vi "Report Plotter.vi"(0 "Plot":refnum<vi>, 1 "Path":refnum<vi>, 2 "Vision Overlay":refnum<vi>, 3 "Indicators":T2, 4 "Play":refnum<vi>, 5 "Exit":refnum<vi>, 7 "Visualized Color Plane":refnum<vi>, 9 "Slider":refnum<vi>, 11 "error in":errorcluster, 12 "Image Indicator":variant, 13 "Loading Bar":refnum<vi>, 14 "Image Type":T1=4 items=["Grayscale (U8)", "Grayscale (I16)", "Grayscale (SGL)", "Complex (CSG)", "RGB (U32)", "HSL (U32)", "RGB (U64)", "Grayscale (U16)"]) -> (15 "error out":errorcluster)   [LabVIEW 2012, in "Report.lvlib"]
uses:
  Report.lvlib
  <vilib>/Waveform/WDTOps.llb/WDT Get XY Value DBL.vi
  <vilib>/Waveform/WDTOps.llb/WDT Number of Waveform Samples DBL.vi
  <vilib>/Utility/xml.llb/Read From XML File(array).vi
  <vilib>/vision/NI_Vision_Development_Module.lvlib
panel:
  out "XML Elements":string[](array[string])
  out "Exit":bool
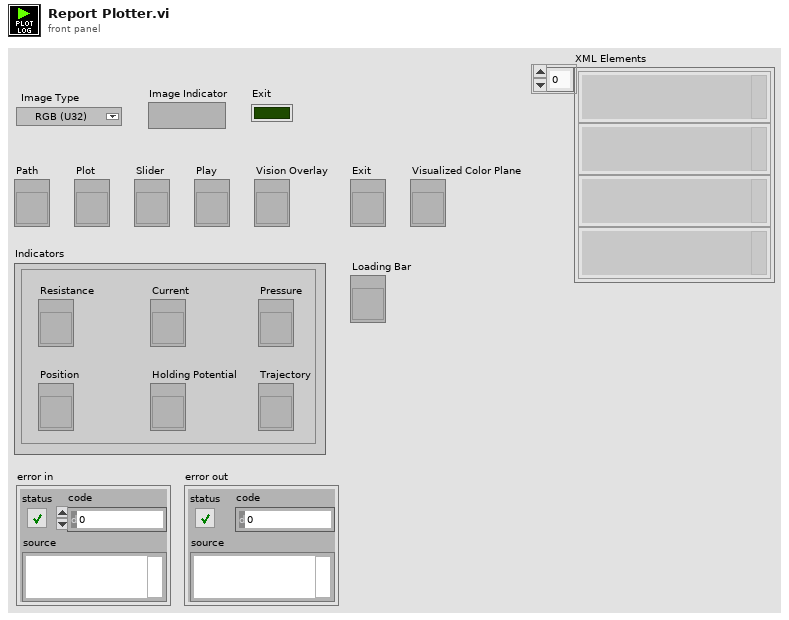
[diagram p1: front panel]
types:
  T1 = typedef "Image Type" = u32
  T2 = cluster{"Resistance":refnum<vi>, "Current":refnum<vi>, "Pressure":refnum<vi>, "Holding Potential":refnum<vi>, "Position":refnum<vi>, "Trajectory":refnum<vi>}
  T3 = cluster{"Name":string, "Color":u32, "Style":u8, "Point Style":u8, "Name Visible":bool, "Allow Drag":bool, "Cursor Mode":u32, "Plot":i32, "Index":i32, "Position":cluster{"X":dbl, "Y":dbl}, "X Scale":u32, "Y Scale":u32, "Watch Plots":i32[], "Watch All Plots":bool, "Plot Area":i32, "Label Offset":cluster{"X":dbl, "Y":dbl}}
  T4 = cluster{"Name":string, "Color":i32, "Style":u8, "Point Style":u8, "Name Visible":bool, "Allow Drag":bool, "Cursor Mode":u32, "Plot":i32, "Index":i32, "Position":cluster{"X":dbl, "Y":dbl}, "X Scale":u32, "Y Scale":u32, "Watch Plots":i32[], "Watch All Plots":bool, "Plot Area":i32, "Label Offset":cluster{"X":dbl, "Y":dbl}}
  T5 = typedef "IMAQ Image.ctl" = refnum<image>
  T6 = cluster{"Name":string, "Color":u32, "Style":u8, "Point Style":u8, "Name Visible":bool, "Allow Drag":bool, "Cursor Mode":u32, "Plot":i32, "Index":i32, "Position":cluster{"X":dbl, "Y":dbl}, "X Scale":u32, "Y Scale":u32, "Watch Plots":i32[], "Watch All Plots":bool, "Plot Area":i32, "Label Offset":cluster{"X":dbl, "Y":dbl}}[]
  T7 = cluster{"Name":string, "Color":i32, "Style":u8, "Point Style":u8, "Name Visible":bool, "Allow Drag":bool, "Cursor Mode":u32, "Plot":i32, "Index":i32, "Position":cluster{"X":dbl, "Y":dbl}, "X Scale":u32, "Y Scale":u32, "Watch Plots":i32[], "Watch All Plots":bool, "Plot Area":i32, "Label Offset":cluster{"X":dbl, "Y":dbl}}[]
  T8 = typedef "LVRangeTypeDef.ctl" = cluster{"Minimum":dbl, "Maximum":dbl, "Increment":dbl, "Minor Increment":dbl, "Start":dbl}
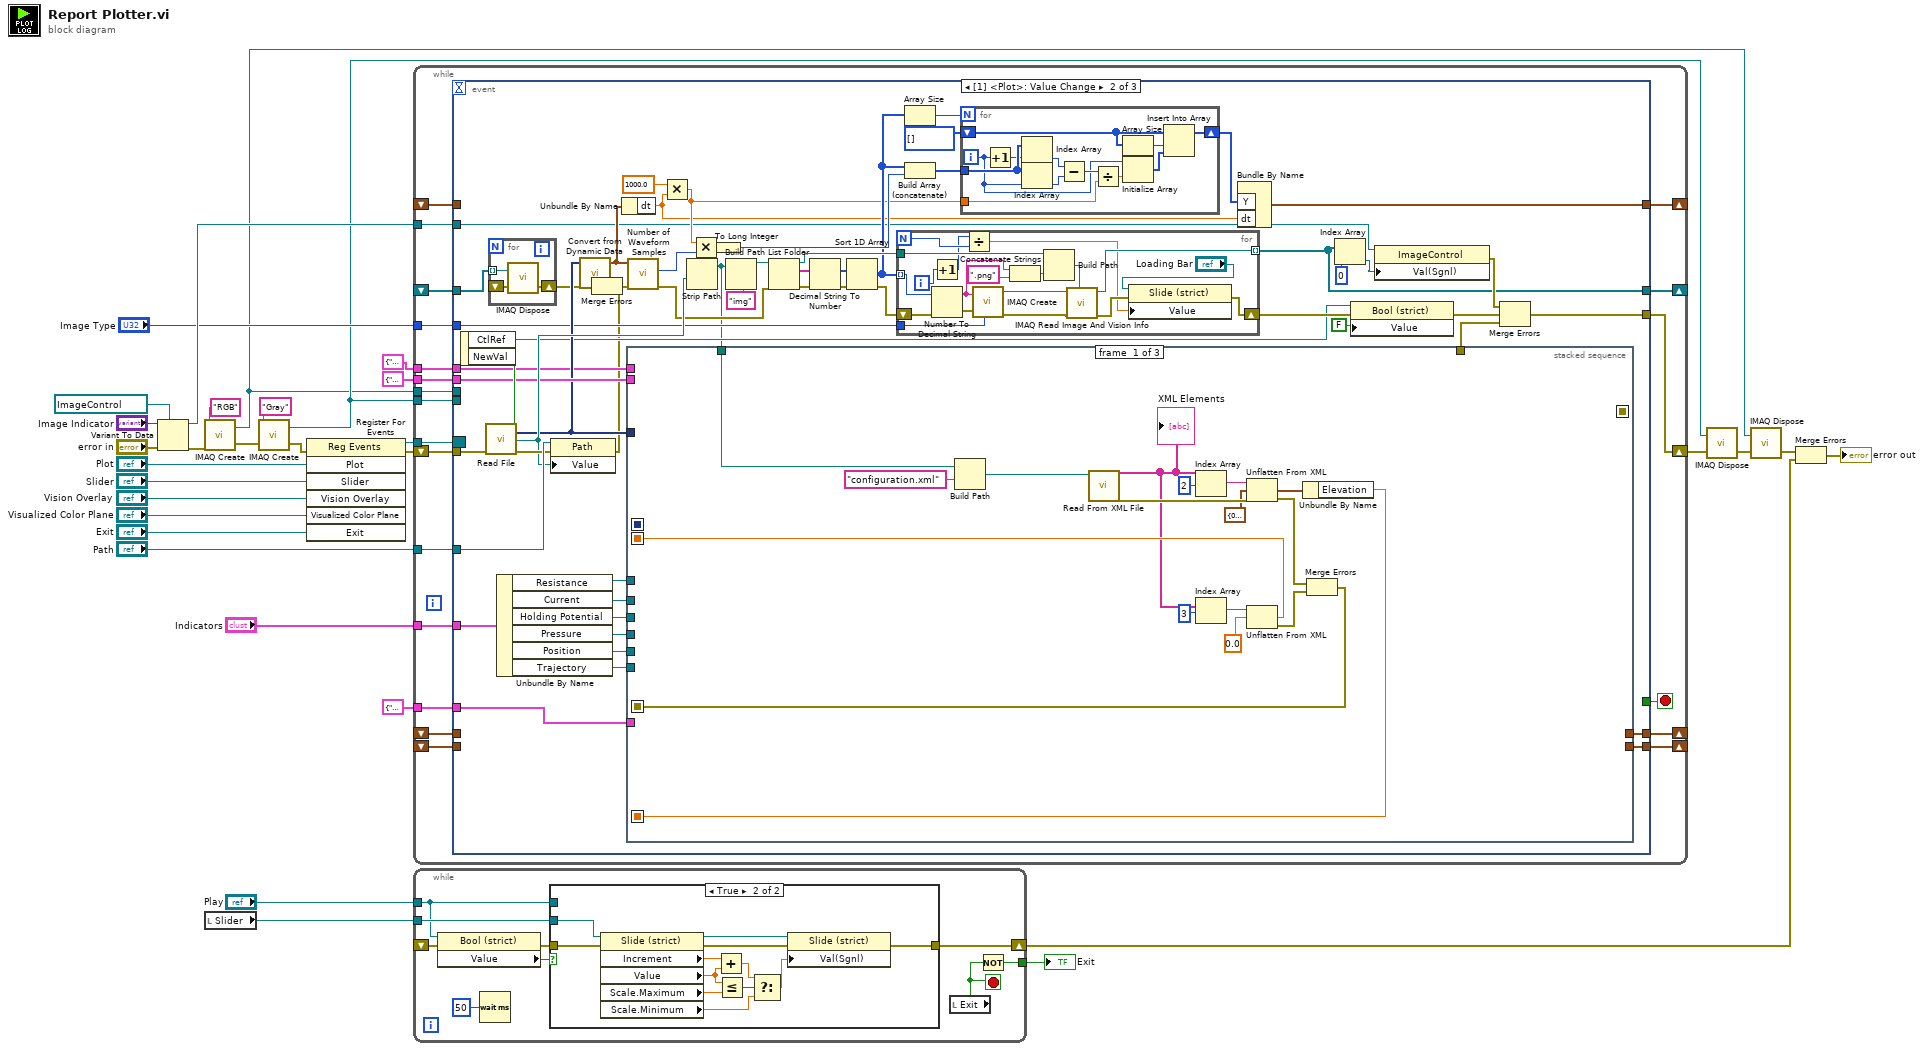
[diagram p0: block diagram]
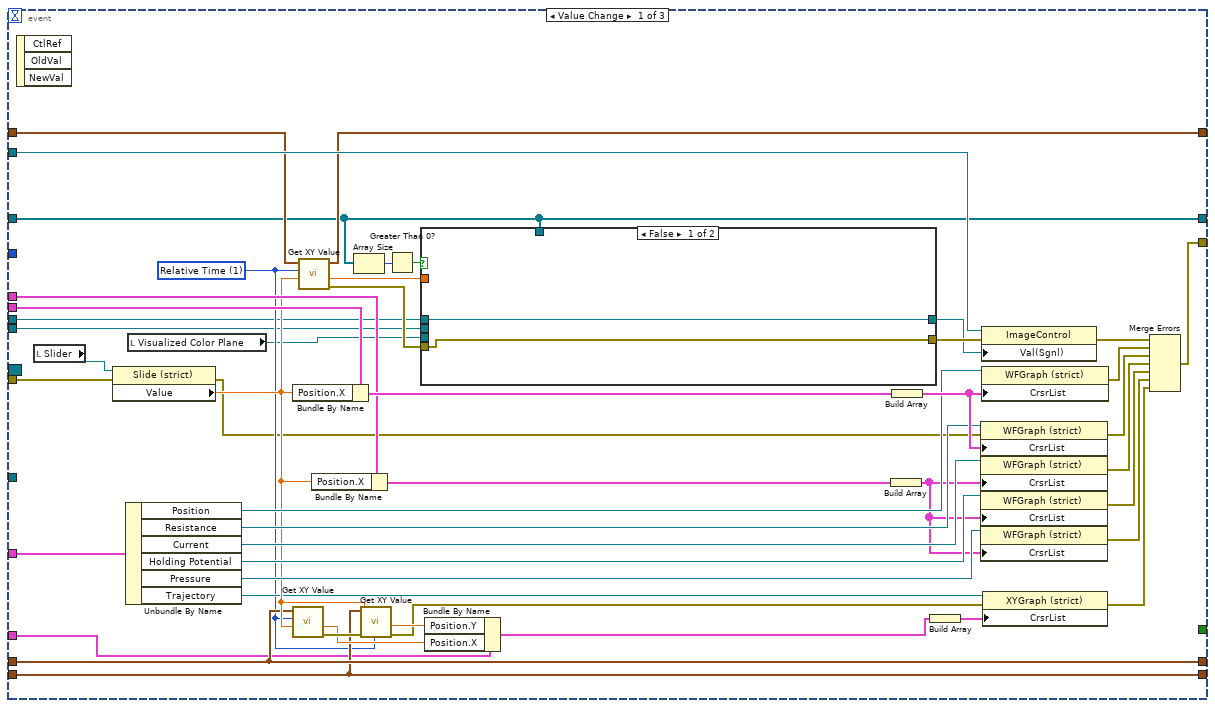
[diagram p3: hidden frame]
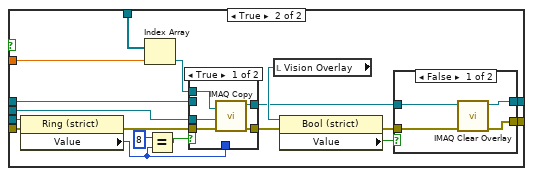
[diagram p4: hidden frame]
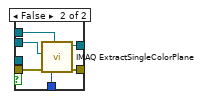
[diagram p5: hidden frame]
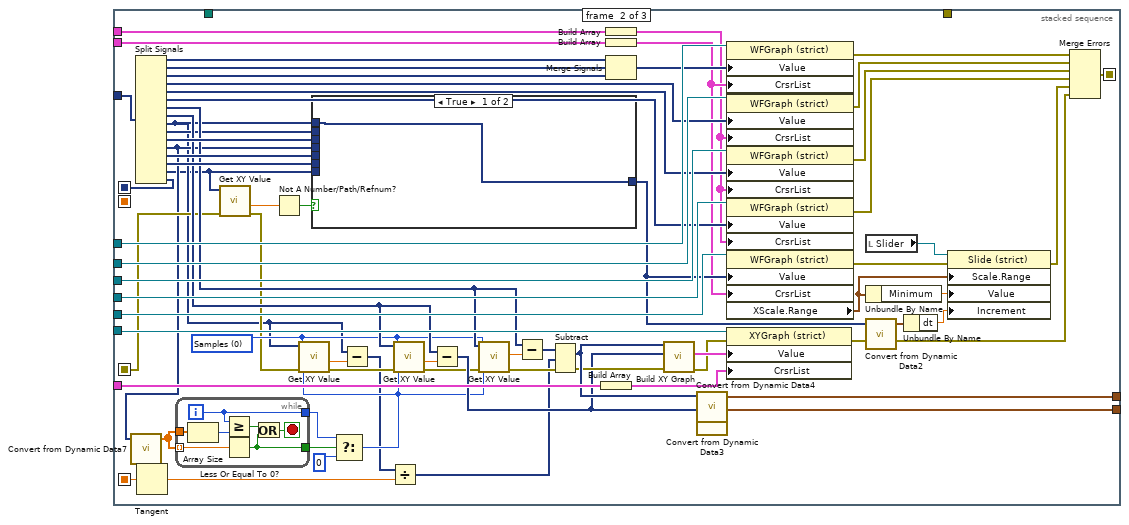
[diagram p7: hidden frame]
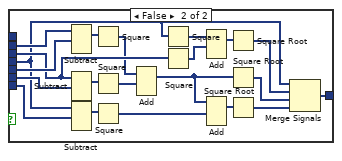
[diagram p8: hidden frame]
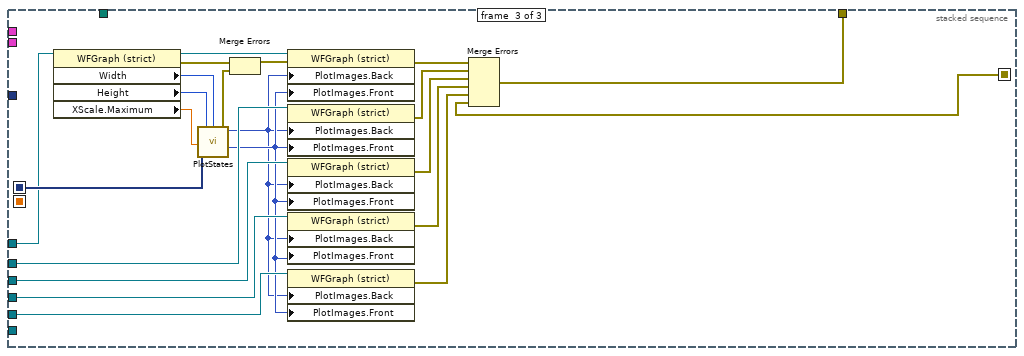
[diagram p9: hidden frame]
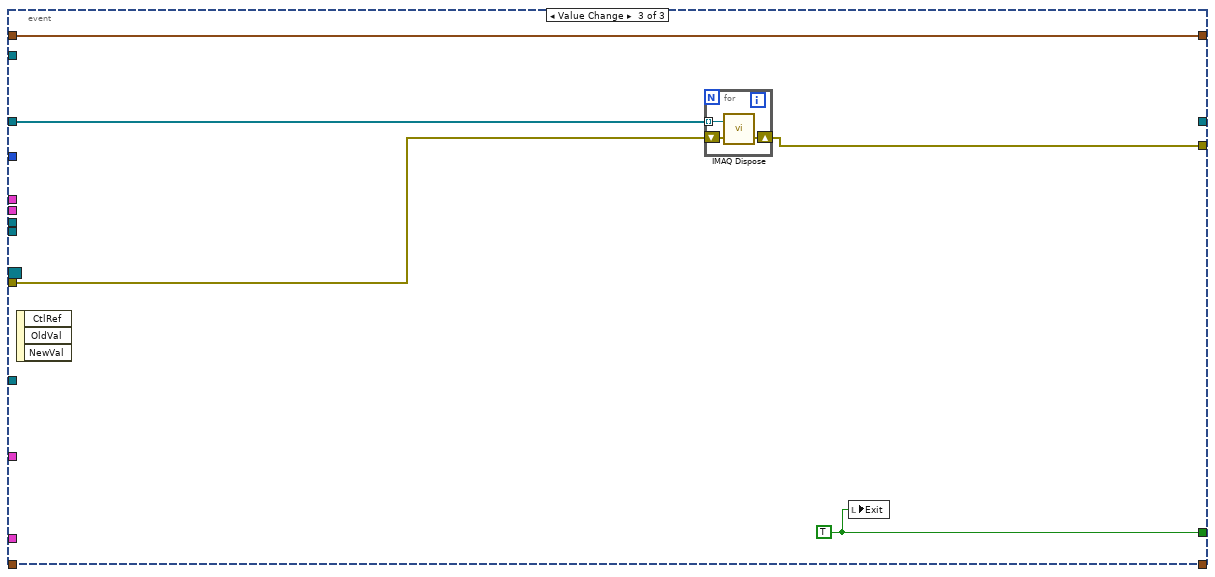
[diagram p10: hidden frame]
diagram:
  n1 = Variant To Data(error in="error in", type=refnum<vi> refnum ("Image"), Variant="Image Indicator") -> (data=w23:refnum<vi>, error out=w13:errorcluster)
  n2 = call "IMAQ Create"("Image Name"="RGB", "error in (no error)"=w13) -> ("New Image"=w1:T5, "error out"=w8:errorcluster)  [unwired: 3 in]
  n3 = local read "Slider"() -> (w18:refnum<vi>)
  n4 = call "IMAQ Create"("Image Name"="Gray", "error in (no error)"=w8) -> ("New Image"=w2:T5, "error out"=w6:errorcluster)  [unwired: 3 in]
  n5 = register-events(error in=w6, "Plot", "Slider", "Vision Overlay", "Visualized Color Plane", "Exit") -> (reference out=w28:refnum<event-registration>, error out=w14:errorcluster)  [unwired: 1 in]
  n6 = while {
    shift-right: [w49] -> w4
    shift-left: w14 -> [w53]
    tunnel: "Indicators" -> [w52]
    tunnel: "Path" -> [w51]
    tunnel: w28 -> [w50]
    tunnel: T4 {"Name"="Cursor", "Color"=16711680, "Style"=2, "Point Style"=2, "Name Visible"=FALSE, "Allow Drag"=TRUE, "Cursor Mode"=2, "Plot"=-1, "Index"=0, "Position"={"X"=0.0, "Y"=0.0}, "X Scale"=0, "Y Scale"=0, "Watch Plots"=[], "Watch All Plots"=TRUE, "Plot Area"=0, "Label Offset"={"X"=0.0, "Y"=0.0}} -> [w48]
    tunnel: T3 {"Name"="Trajectory", "Color"=16711680, "Style"=8, "Point Style"=8, "Name Visible"=FALSE, "Allow Drag"=TRUE, "Cursor Mode"=0, "Plot"=0, "Index"=0, "Position"={"X"=0.0, "Y"=0.0}, "X Scale"=0, "Y Scale"=0, "Watch Plots"=[], "Watch All Plots"=FALSE, "Plot Area"=0, "Label Offset"={"X"=0.1, "Y"=10.0}} ("element") -> [w47]
    shift-right: [w46] -> _
    shift-left: _ -> [w45]
    tunnel: w23 -> [w44]
    shift-right: [w43] -> _
    shift-left: _ -> [w42]
    tunnel: "Image Type" -> [w41]
    tunnel: T3 {"Name"="Cursor 0", "Color"=16711680, "Style"=2, "Point Style"=2, "Name Visible"=FALSE, "Allow Drag"=TRUE, "Cursor Mode"=1, "Plot"=-1, "Index"=0, "Position"={"X"=0.0, "Y"=0.0}, "X Scale"=0, "Y Scale"=0, "Watch Plots"=[], "Watch All Plots"=FALSE, "Plot Area"=0, "Label Offset"={"X"=0.0, "Y"=25.31645569620254}} -> [w40]
    shift-right: [w39] -> _
    shift-left: _ -> [w38]
    shift-right: [w37] -> _
    shift-left: _ -> [w36]
    tunnel: w1 -> [w34]
    tunnel: w2 -> [w33]
    stop <- w35 stop-if-true
    n7 = event shown="[1] <Plot>: Value Change" {
      selector: w50 -> [_ _ _]
      dyn-events: _ -> [_ _ _]
      timeout: _ -> [_ _ _]
      tunnel: w53 -> [w93 w193 w368]
      tunnel: w52 -> [w101 w192 _]
      tunnel: w51 -> [_ w191 _]
      tunnel: [w74 w171 w367] -> w49
      tunnel: w48 -> [w92 w174 _]
      tunnel: w47 -> [w65 w180 _]
      tunnel: [w82 w159 w371] -> w46
      tunnel: w45 -> [w83 _ w371]
      tunnel: w44 -> [w86 w144 _]
      tunnel: [w57 w149 _] -> w43
      tunnel: w42 -> [w57 w142 w369]
      tunnel: w41 -> [_ w158 _]
      tunnel: w40 -> [w79 w153 _]
      tunnel: [w67 w152 _] -> w39
      tunnel: w38 -> [w67 _ _]
      tunnel: [w66 w151 _] -> w37
      tunnel: w36 -> [w66 _ _]
      tunnel: [_ _ w370] -> w35
      tunnel: w34 -> [w59 _ _]
      tunnel: w33 -> [w58 _ _]
      event Value Change {
        w64 = u16 1 items=["Samples", "Relative Time"] ("Y position format")
        n8 = event-data() -> ()  [unwired: 1 in, 3 out]
        n9 = local read "Slider"() -> (w87:refnum<vi>)
        n10 = property class="Slide (strict)"(reference=w87, error in=w93) -> (error out=w56:errorcluster, "Value"=w78:dbl)  [unwired: 1 out]
        n11 = Unbundle By Name(w101) -> ("Position"=w88:refnum<vi>, "Resistance"=w89:refnum<vi>, "Current"=w100:refnum<vi>, "Holding Potential"=w99:refnum<vi>, "Pressure"=w98:refnum<vi>, "Trajectory"=w75:refnum<vi>)
        n12 = local read "Visualized Color Plane"() -> (w60:refnum<vi>)
        n13 = Bundle By Name(cluster=w92, "Position.X"=w78) -> (w91:T4)
        n14 = call-poly <vilib>:"Get XY Value.vi"("Y position"=w78, "Y position format"=w64, "waveform in"=w67) -> ("error out"=w72:errorcluster, "Y value"=w71:dbl)  [unwired: 4 in, 3 out]
        n15 = call-poly <vilib>:"Get XY Value.vi"("Y position"=w78, "Y position format"=w64, "waveform in"=w83) -> ("error out"=w61:errorcluster, "Y value"=w84:dbl, "waveform out"=w82:waveform(dbl))  [unwired: 4 in, 2 out]
        n16 = Bundle By Name(cluster=w79, "Position.X"=w78) -> (w80:T3)
        n17 = Array Size(array=w57) -> (size(s)=w55:i32)
        n18 = call-poly <vilib>:"Get XY Value.vi"("error in (no error)"=w72, "Y position"=w78, "Y position format"=w64, "waveform in"=w66) -> ("error out"=w69:errorcluster, "Y value"=w70:dbl)  [unwired: 3 in, 3 out]
        n19 = Greater Than 0?(x=w55) -> (x > 0?=w54:bool)
        n20 = case shown="False" w54 {
          tunnel: w84 -> [_ w121]
          tunnel: [w103 w120] -> w63
          tunnel: [w102 w119] -> w62
          tunnel: w61 -> [w103 w114]
          tunnel: w60 -> [_ w113]
          tunnel: w59 -> [w102 w107]
          tunnel: w58 -> [_ w105]
          tunnel: w57 -> [_ w104]
          frame False {
          }
          frame True {
            n21 = property on="Property Node" class="Ring (strict)"(reference=w113, error in=w114) -> (error out=w112:errorcluster, "Value"=w108:i32)  [unwired: 1 out]
            n22 = Index Array(array=w104, index=w121) -> (element=w110:T5)
            n23 = Equal?(x=8, y=w108) -> (x = y?=w111:bool)
            n24 = case shown="True" w111 {
              tunnel: w110 -> [w124 w132]
              tunnel: [w126 w131] -> w109
              tunnel: w107 -> [_ w130]
              tunnel: [w125 w129] -> w106
              tunnel: w108 -> [_ w128]
              tunnel: w112 -> [w123 w127]
              tunnel: w105 -> [w122 _]
              frame True {
                n25 = call "IMAQ Copy"("error in (no error)"=w123, "Image Dst"=w122, "Image Src"=w124) -> ("error out"=w125:errorcluster, "Image Dst Out"=w126:T5)  [unwired: 3 in]
              }
              frame False {
                n26 = call "IMAQ ExtractSingleColorPlane"("Color Plane"=w128, "error in (no error)"=w127, "Image Dst"=w130, "Image Src"=w132) -> ("error out"=w129:errorcluster, "Image Dst Out"=w131:T5)  [unwired: 6 in]
              }
            }
            n27 = local read "Vision Overlay"() -> (w117:refnum<vi>)
            n28 = property class="Bool (strict)"(reference=w117, error in=w106) -> (error out=w118:errorcluster, "Value"=w116:bool)  [unwired: 1 out]
            n29 = case shown="False" w116 {
              tunnel: [w136 w138] -> w120
              tunnel: w118 -> [w133 w138]
              tunnel: [w135 w137] -> w119
              tunnel: w109 -> [w134 w137]
              frame False {
                n30 = call "IMAQ Clear Overlay"("error in (no error)"=w133, "Image"=w134) -> ("error out"=w136:errorcluster, "Image Out"=w135:T5)  [unwired: 8 in]
              }
              frame True {
              }
            }
          }
        }
        n31 = Bundle By Name(cluster=w65, "Position.Y"=w70, "Position.X"=w71) -> (w77:T3)
        n32 = Build Array(w80) -> (w81:T6)
        n33 = Build Array(w91) -> (w90:T7)
        n34 = Build Array(w77) -> (w76:T6)
        n35 = property class="WFGraph (strict)"(reference=w89, error in=w56, "CrsrList"=w90) -> (error out=w97:errorcluster)  [unwired: 1 out]
        n36 = property class="WFGraph (strict)"(reference=w100, "CrsrList"=w81) -> (error out=w96:errorcluster)  [unwired: 1 in, 1 out]
        n37 = property class="WFGraph (strict)"(reference=w99, "CrsrList"=w81) -> (error out=w95:errorcluster)  [unwired: 1 in, 1 out]
        n38 = property class="WFGraph (strict)"(reference=w98, "CrsrList"=w81) -> (error out=w94:errorcluster)  [unwired: 1 in, 1 out]
        n39 = property class="ImageControl"(reference=w86, error in=w63, "Val(Sgnl)"=w62) -> (error out=w85:errorcluster)  [unwired: 1 out]
        n40 = property class="WFGraph (strict)"(reference=w88, "CrsrList"=w90) -> (error out=w73:errorcluster)  [unwired: 1 in, 1 out]
        n41 = property on="Property Node" class="XYGraph (strict)"(reference=w75, error in=w69, "CrsrList"=w76) -> (error out=w68:errorcluster)  [unwired: 1 out]
        n42 = Merge Errors(w85, w73, w97, w96, w95, w94, w68) -> (w74:errorcluster)
      }
      event Value Change {
        n43 = event-data() -> ("CtlRef"=w160:refnum<vi>, "NewVal"=w183:bool)  [unwired: 1 in]
        n44 = call "Read File"("error in (no error)"=w193, "Reset"=w183) -> ("error out"=w181:errorcluster, "Filename Out"=w179:path, "Signals"=w170:dynamicdata)  [unwired: 4 in, 3 out]
        n45 = for {
          tunnel: w142 -> [w196] mode=indexing
          shift-right: [w194] -> w139
          shift-left: _ -> [w195]
          n46 = call "IMAQ Dispose"("Image"=w196, "error in (no error)"=w195) -> ("error out"=w194:errorcluster)  [unwired: 4 in]
        }
        n47 = Unbundle By Name(w192) -> ("Resistance"=w190:refnum<vi>, "Current"=w189:refnum<vi>, "Holding Potential"=w188:refnum<vi>, "Pressure"=w187:refnum<vi>, "Position"=w186:refnum<vi>, "Trajectory"=w184:refnum<vi>)
        n48 = property class="Path"(reference=w191, error in=w181, "Value"=w179) -> (error out=w141:errorcluster)  [unwired: 1 out]
        n49 = call "Convert from Dynamic Data"("Dynamic Data Type"=w170) -> ("Waveform"=w169:waveform(dbl))  [unwired: 3 in]
        n50 = Merge Errors(w139, w141) -> (w140:errorcluster)
        n51 = Unbundle By Name(w169) -> ("dt"=w146:dbl)
        n52 = call-poly <vilib>:"Number of Waveform Samples.vi"("error in (no error)"=w140, "waveform in"=w169) -> ("error out"=w163:errorcluster, "number of samples"=w165:i32)  [unwired: 7 in, 1 out]
        n53 = Multiply(x=1000.0 ("y"), y=w146) -> (x*y=w164:dbl)
        n54 = Strip Path(path=w179) -> (stripped path=w143:path)  [unwired: 1 out]
        n55 = stacked-sequence {
          seq-local: [_ w278 _] -> [_ _ w366]
          seq-local: [_ w306 _] -> [_ _ w347]
          seq-local: [w240 _ _] -> [_ w274 _]
          seq-local: [w243 _ _] -> [_ _ _]
          seq-local: [w242 _ _] -> [_ w248 _]
          tunnel: w170 -> [_ w305 _]
          tunnel: w190 -> [_ w314 w356]
          tunnel: w189 -> [_ w313 w364]
          tunnel: w188 -> [_ w312 w363]
          tunnel: w187 -> [_ w311 w362]
          tunnel: w186 -> [_ w298 w361]
          tunnel: [_ _ w348] -> w185
          tunnel: w184 -> [_ w299 _]
          tunnel: w174 -> [_ w293 _]
          tunnel: w180 -> [_ w292 _]
          tunnel: w153 -> [_ w284 _]
          tunnel: [_ w281 _] -> w152
          tunnel: [_ w280 _] -> w151
          tunnel: w143 -> [w241 _ _]
          frame #0 {
            n56 = Build Path(base path=w241, name or relative path="configuration.xml") -> (appended path=w230:path)
            n57 = call-poly <vilib>:"Read From XML File.vi"("XML File Path"=w230) -> ("error out"=w238:errorcluster, "XML Elements"=w234:string[])  [unwired: 8 in, 1 out]
            "XML Elements" <- w234
            n58 = Index Array(array=w234, index=2) -> (element=w237:string)
            n59 = Index Array(array=w234, index=3) -> (element=w236:string)
            n60 = Unflatten From XML(xml string=w237, type=cluster{"Azimut":dbl, "Elevation":dbl} {"Azimut"=0.0, "Elevation"=0.0} ("Angles"), error in (no error)=w238) -> (value=w227:cluster{"Azimut":dbl, "Elevation":dbl}, error out=w233:errorcluster)
            n61 = Unflatten From XML(xml string=w236, type=0.0 ("Surface Manip")) -> (value=w243:dbl, error out=w232:errorcluster)  [unwired: 1 in]
            n62 = Unbundle By Name(w227) -> ("Elevation"=w240:dbl)
            n63 = Merge Errors(w233, w232) -> (w242:errorcluster)
          }
          frame #1 {
            w258 = u16 0 items=["Samples", "Relative Time"] ("Y position format")
            n64 = Split Signals(w305) -> (w290:dynamicdata, w315:dynamicdata, w304:dynamicdata, w301:dynamicdata, w302:dynamicdata, w303:dynamicdata, w259:dynamicdata, w260:dynamicdata, w245:dynamicdata, w250:dynamicdata, w261:dynamicdata, w246:dynamicdata, w262:dynamicdata, w263:dynamicdata, w244:dynamicdata, w278:dynamicdata)  [unwired: 16 in]
            n65 = call "Convert from Dynamic Data7"("Dynamic Data Type"=w246) -> ("Array"=w264:dbl[])  [unwired: 3 in]
            n66 = Tangent(1:w274) -> (0:w277:dbl)
            n67 = while {
              tunnel: w264 -> [w344] mode=indexing
              tunnel: w264 -> [w343]
              tunnel: [w341] -> w266
              tunnel: [w338] -> w265
              i -> [w341]
              stop <- w340 stop-if-true
              n68 = Array Size(array=w343) -> (size(s)=w342:i32)
              n69 = Greater Or Equal?(x=w341, y=w342) -> (x >= y?=w339:bool)
              n70 = Less Or Equal To 0?(x=w344) -> (x <= 0?=w338:bool)
              n71 = Or(x=w339, y=w338) -> (x .or. y?=w340:bool)
            }
            n72 = call-poly <vilib>:"Get XY Value.vi"("error in (no error)"=w248, "waveform in"=w244) -> ("error out"=w247:errorcluster, "Y value"=w251:dbl)  [unwired: 5 in, 3 out]
            n73 = Not A Number/Path/Refnum?(number/path/refnum=w251) -> (NaN/Path/Refnum?=w249:bool)
            n74 = case shown="True" w249 {
              tunnel: [w316 w337] -> w289
              tunnel: w244 -> [_ w332]
              tunnel: w263 -> [_ w331]
              tunnel: w262 -> [_ w330]
              tunnel: w261 -> [_ w326]
              tunnel: w250 -> [_ w318]
              tunnel: w246 -> [_ w317]
              tunnel: w245 -> [w316 _]
              frame True {
              }
              frame False {
                n75 = Subtract(1:w330, 2:w318) -> (0:w329:dynamicdata)  [unwired: 1 in, 1 out]
                n76 = Subtract(1:w331, 2:w326) -> (0:w328:dynamicdata)  [unwired: 1 in, 1 out]
                n77 = Subtract(1:w332, 2:w317) -> (0:w327:dynamicdata)  [unwired: 1 in, 1 out]
                n78 = Square(x=w329) -> (x^2=w325:dynamicdata)
                n79 = Square(x=w328) -> (x^2=w324:dynamicdata)
                n80 = Square(x=w327) -> (x^2=w323:dynamicdata)
                n81 = Add(1:w324, 2:w325) -> (0:w322:dynamicdata)  [unwired: 1 in, 1 out]
                n82 = Square(x=w317) -> (x^2=w335:dynamicdata)
                n83 = Square(x=w326) -> (x^2=w334:dynamicdata)
                n84 = Add(1:w334, 2:w335) -> (0:w336:dynamicdata)  [unwired: 1 in, 1 out]
                n85 = Add(1:w323, 2:w322) -> (0:w321:dynamicdata)  [unwired: 1 in, 1 out]
                n86 = Square Root(x=w336) -> (sqrt(x)=w333:dynamicdata)
                n87 = Square Root(x=w322) -> (sqrt(x)=w320:dynamicdata)
                n88 = Square Root(x=w321) -> (sqrt(x)=w319:dynamicdata)
                n89 = Merge Signals(w317, w333, w320, w319) -> (w337:dynamicdata)
              }
            }
            n90 = Select(t=w266, s=w265, f=0 ("t")) -> (s? t:f=w255:i32)
            n91 = call-poly <vilib>:"Get XY Value.vi"("error in (no error)"=w247, "Y position"=w255, "Y position format"=w258, "waveform in"=w245) -> ("error out"=w257:errorcluster, "Y value"=w256:dbl)  [unwired: 3 in, 3 out]
            n92 = Subtract(x=w245, y=w256) -> (x-y=w253:dynamicdata)
            n93 = Divide(x=w253, y=w277) -> (x/y=w252:dynamicdata)
            n94 = call-poly <vilib>:"Get XY Value.vi"("error in (no error)"=w257, "Y position"=w255, "Y position format"=w258, "waveform in"=w260) -> ("error out"=w268:errorcluster, "Y value"=w276:dbl)  [unwired: 3 in, 3 out]
            n95 = Subtract(x=w260, y=w276) -> (x-y=w269:dynamicdata)
            n96 = call-poly <vilib>:"Get XY Value.vi"("error in (no error)"=w268, "Y position"=w255, "Y position format"=w258, "waveform in"=w259) -> ("error out"=w270:errorcluster, "Y value"=w275:dbl)  [unwired: 3 in, 3 out]
            n97 = Subtract(x=w259, y=w275) -> (x-y=w254:dynamicdata)
            n98 = Subtract(1:w252, 2:w254, 4:w270) -> (0:w273:dynamicdata, 3:w271:errorcluster)
            n99 = Build Array(w292) -> (w291:T6)
            n100 = Build Array(w284) -> (w282:T6)
            n101 = Build Array(w293) -> (w283:T7)
            n102 = Merge Signals(w290, w315, w304) -> (w300:dynamicdata)
            n103 = call "Build XY Graph"("error in (no error)"=w271, "Y Input"=w269, "X Input"=w273) -> ("error out"=w272:errorcluster, "XY Graph"=w279:cluster{"Y":dbl[], "Y":dbl[]}[])  [unwired: 2 in, 5 out]
            n104 = call "Convert from Dynamic Data4"("Dynamic Data Type"=w273) -> ("Waveform"=w281:waveform(dbl))  [unwired: 3 in]
            n105 = call "Convert from Dynamic Data3"("Dynamic Data Type"=w269) -> ("Waveform"=w280:waveform(dbl))  [unwired: 3 in]
            n106 = property class="WFGraph (strict)"(reference=w314, "Value"=w300, "CrsrList"=w283) -> (error out=w310:errorcluster)  [unwired: 1 in, 1 out]
            n107 = property class="WFGraph (strict)"(reference=w313, "Value"=w301, "CrsrList"=w282) -> (error out=w309:errorcluster)  [unwired: 1 in, 1 out]
            n108 = property class="WFGraph (strict)"(reference=w312, "Value"=w302, "CrsrList"=w282) -> (error out=w308:errorcluster)  [unwired: 1 in, 1 out]
            n109 = property class="WFGraph (strict)"(reference=w311, "Value"=w303, "CrsrList"=w282) -> (error out=w307:errorcluster)  [unwired: 1 in, 1 out]
            n110 = property class="WFGraph (strict)"(reference=w298, "Value"=w289, "CrsrList"=w283) -> (error out=w297:errorcluster, "XScale.Range"=w294:T8)  [unwired: 1 in, 1 out]
            n111 = property class="XYGraph (strict)"(reference=w299, error in=w272, "Value"=w279, "CrsrList"=w291) -> (error out=w295:errorcluster)  [unwired: 1 out]
            n112 = local read "Slider"() -> (w288:refnum<vi>)
            n113 = Unbundle By Name(w294) -> ("Minimum"=w287:dbl)
            n114 = call "Convert from Dynamic Data2"("Dynamic Data Type"=w289) -> ("Waveform"=w286:waveform(dbl))  [unwired: 3 in]
            n115 = Unbundle By Name(w286) -> ("dt"=w285:dbl)
            n116 = property class="Slide (strict)"(reference=w288, error in=w297, "Scale.Range"=w294, "Value"=w287, "Increment"=w285) -> (error out=w296:errorcluster)  [unwired: 1 out]
            n117 = Merge Errors(w310, w309, w308, w307, w296, w295) -> (w306:errorcluster)
          }
          frame #2 {
            n118 = property class="WFGraph (strict)"(reference=w356) -> (reference out=w357:refnum<vi>, error out=w355:errorcluster, "Width"=w358:u32, "Height"=w359:u32, "XScale.Maximum"=w360:dbl)  [unwired: 1 in]
            n119 = call "PlotStates.vi"("Width"=w358, "Height"=w359, "XScale.Max"=w360, "waveform in"=w366) -> ("error out"=w365:errorcluster, "Middle"=w346:picture, "Back"=w345:picture)  [unwired: 5 in]
            n120 = Merge Errors(w355, w365) -> (w349:errorcluster)
            n121 = property class="WFGraph (strict)"(reference=w357, error in=w349, "PlotImages.Back"=w345, "PlotImages.Front"=w346) -> (error out=w354:errorcluster)  [unwired: 1 out]
            n122 = property class="WFGraph (strict)"(reference=w364, "PlotImages.Back"=w345, "PlotImages.Front"=w346) -> (error out=w353:errorcluster)  [unwired: 1 in, 1 out]
            n123 = property class="WFGraph (strict)"(reference=w363, "PlotImages.Back"=w345, "PlotImages.Front"=w346) -> (error out=w352:errorcluster)  [unwired: 1 in, 1 out]
            n124 = property class="WFGraph (strict)"(reference=w362, "PlotImages.Back"=w345, "PlotImages.Front"=w346) -> (error out=w351:errorcluster)  [unwired: 1 in, 1 out]
            n125 = property class="WFGraph (strict)"(reference=w361, "PlotImages.Back"=w345, "PlotImages.Front"=w346) -> (error out=w350:errorcluster)  [unwired: 1 in, 1 out]
            n126 = Merge Errors(w354, w353, w352, w351, w350, w347) -> (w348:errorcluster)
          }
        }
        n127 = Multiply(x=w164, y=w165) -> (x*y=w166:dbl)
        n128 = To Long Integer(number=w166) -> (32bit integer=w168:i32)
        n129 = Build Path(base path=w143, name or relative path="img") -> (appended path=w177:path)
        n130 = List Folder(path=w177, error in=w163) -> (path out=w172:path, filenames=w176:string[], error out=w173:errorcluster)  [unwired: 3 out]
        n131 = Decimal String To Number(string=w176) -> (number=w175:i32[])  [unwired: 2 in, 1 out]
        n132 = Sort 1D Array(array=w175) -> (sorted array=w167:i32[])
        n133 = for {
          N -> [w215]
          tunnel: w167 -> [w216] mode=indexing
          tunnel: [w218] -> w149 mode=indexing
          shift-right: [w213] -> w162
          shift-left: w173 -> [w226]
          tunnel: w172 -> [w225]
          tunnel: w158 -> [w221]
          i -> [w210]
          n134 = Increment(x=w210) -> (x+1=w209:i32)
          n135 = Number To Decimal String(number=w216) -> (decimal integer string=w222:string)  [unwired: 1 in]
          n136 = Divide(x=w209, y=w215) -> (x/y=w212:dbl)
          n137 = call "IMAQ Create"("Image Name"=w222, "Image Type"=w221, "error in (no error)"=w226) -> ("New Image"=w220:T5, "error out"=w219:errorcluster)  [unwired: 1 in, 1 out]
          n138 = Concatenate Strings(w222, ".png" ("string")) -> (w223:string)
          n139 = Build Path(base path=w225, name or relative path=w223) -> (appended path=w217:path)
          n140 = call "IMAQ Read Image And Vision Info"("File Path"=w217, "error in (no error)"=w219, "Image"=w220) -> ("error out"=w214:errorcluster, "Image Out"=w218:T5)  [unwired: 6 in, 1 out]
          n141 = property class="Slide (strict)"(reference="Loading Bar", error in=w214, "Value"=w212) -> (error out=w213:errorcluster)  [unwired: 1 out]
        }
        n142 = Array Size(array=w167) -> (size(s)=w157:i32)
        n143 = Build Array (concatenate)(w167, w168) -> (w155:i32[])
        n144 = for {
          N: w157 -> [_]
          tunnel: w155 -> [w208]
          shift-right: [w204] -> w154
          shift-left: i32[] [] -> [w203]
          tunnel: w164 -> [w199]
          i -> [w197]
          n145 = Increment(x=w197) -> (x+1=w207:i32)
          n146 = Index Array(array=w208, index=w207) -> (element=w206:i32)
          n147 = Index Array(array=w208, index=w197) -> (element=w201:i32)
          n148 = Subtract(x=w206, y=w201) -> (x-y=w200:i32)
          n149 = Divide(x=w200, y=w199) -> (x/y=w198:dbl)
          n150 = Array Size(array=w203) -> (size(s)=w202:i32)
          n151 = Initialize Array(w197, w198) -> (w205:i32[])
          n152 = Insert Into Array(array=w203, index=w202, new element=w205) -> (w204:i32[])
        }
        n153 = Bundle By Name("Y"=w154, "dt"=w146) -> (w159:waveform(i32))  [unwired: 1 in]
        n154 = Index Array(array=w149, index=0) -> (element=w147:T5)
        n155 = property class="Bool (strict)"(reference=w160, error in=w162, "Value"=FALSE) -> (error out=w161:errorcluster)  [unwired: 1 out]
        n156 = property class="ImageControl"(reference=w144, "Val(Sgnl)"=w147) -> (error out=w150:errorcluster)  [unwired: 1 in, 1 out]
        n157 = Merge Errors(w150, w161, w185) -> (w171:errorcluster)
      }
      event Value Change {
        w370 = TRUE
        n158 = event-data() -> ()  [unwired: 1 in, 3 out]
        n159 = for {
          tunnel: w369 -> [w374] mode=indexing
          shift-right: [w372] -> w367
          shift-left: w368 -> [w373]
          n160 = call "IMAQ Dispose"("Image"=w374, "error in (no error)"=w373) -> ("error out"=w372:errorcluster)  [unwired: 4 in]
        }
        n161 = local write "Exit"(w370) -> ()
      }
    }
  }
  n162 = while {
    tunnel: "Play" -> [w379]
    shift-right: [w383] -> w16
    shift-left: _ -> [w381]
    tunnel: w18 -> [w382]
    tunnel: [w377] -> w15
    stop <- w375 stop-if-true
    n163 = property class="Bool (strict)"(reference=w379, error in=w381) -> (error out=w380:errorcluster, "Value"=w378:bool)  [unwired: 1 out]
    n164 = Wait (ms)(milliseconds to wait=u32 50) -> ()  [unwired: 1 out]
    n165 = case shown="True" w378 {
      tunnel: w379 -> [_ _]
      tunnel: [w384 w385] -> w383
      tunnel: w380 -> [w384 w396]
      tunnel: w382 -> [_ w395]
      frame False {
      }
      frame True {
        n166 = property class="Slide (strict)"(reference=w395, error in=w396) -> (reference out=w394:refnum<vi>, error out=w393:errorcluster, "Increment"=w388:dbl, "Value"=w392:dbl, "Scale.Maximum"=w391:dbl, "Scale.Minimum"=w389:dbl)
        n167 = Add(x=w388, y=w392) -> (x+y=w387:dbl)
        n168 = Less Or Equal?(x=w392, y=w391) -> (x <= y?=w390:bool)
        n169 = Select(t=w387, s=w390, f=w389) -> (s? t:f=w386:dbl)
        n170 = property class="Slide (strict)"(reference=w394, error in=w393, "Val(Sgnl)"=w386) -> (error out=w385:errorcluster)  [unwired: 1 out]
      }
    }
    n171 = local read "Exit"() -> (w375:bool)
    n172 = Not(x=w375) -> (.not. x?=w377:bool)
  }
  "Exit" <- w15
  n173 = call "IMAQ Dispose"("Image"=w2, "error in (no error)"=w4) -> ("error out"=w5:errorcluster)  [unwired: 4 in]
  n174 = call "IMAQ Dispose"("Image"=w1, "error in (no error)"=w5) -> ("error out"=w3:errorcluster)  [unwired: 4 in]
  n175 = Merge Errors(w3, w16) -> (→"error out":errorcluster)
